vi "Read Lang LUT.vi"(8 "error in (no error)":errorcluster, 11 "Resource Data in":refnum<class "Resource Data.lvclass">) -> (0 "error out":errorcluster, 2 "Lang LUT":variant, 3 "Resource Data out":refnum<class "Resource Data.lvclass">)   [LabVIEW 2013, in "SET Project Data.lvlib" / "Resource Data.lvclass"]
uses:
  Resource Data.lvclass
  Resource Data.lvclass/Resource Data.ctl
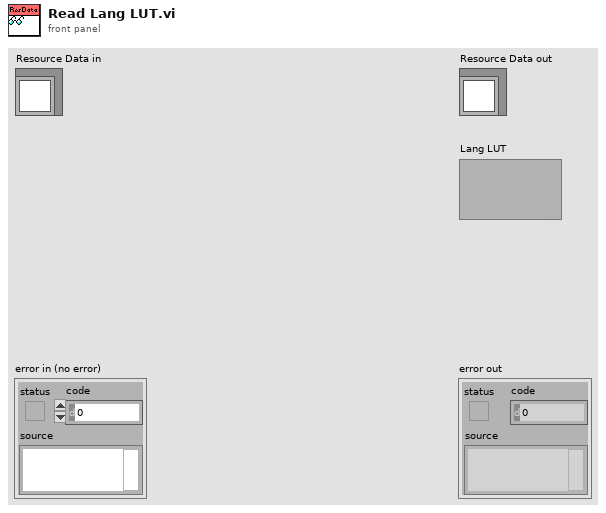
[diagram p1: front panel]
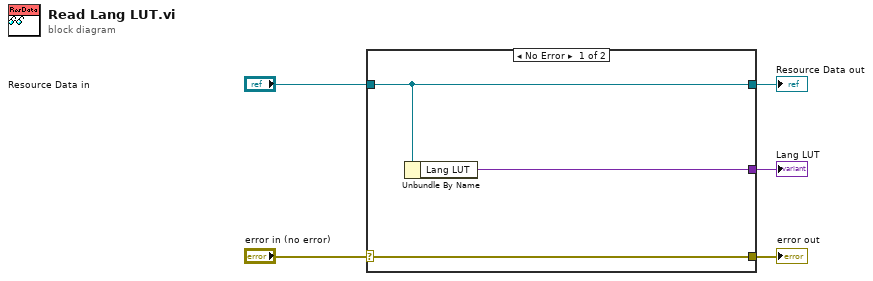
[diagram p0: block diagram]
diagram:
  n1 = case shown="No Error" "error in (no error)" {
    selector: "error in (no error)" -> [w8 w9]
    tunnel: [w8 w9] -> w4
    tunnel: [w7 w10] -> w2
    tunnel: "Resource Data in" -> [w7 w10]
    tunnel: [w6 _] -> w1
    frame No Error {
      n2 = Unbundle By Name(w7) -> ("Lang LUT"=w6:variant)
    }
    frame Error {
    }
  }
  "error out" <- w4
  "Resource Data out" <- w2
  "Lang LUT" <- w1
